vi "Save last shot data.vi"() -> ()   [LabVIEW 2015]
uses:
  Shot data.ctl
  <vilib>/Utility/config.llb/Write Key (I32).vi
  <vilib>/Utility/config.llb/Write Key (String).vi
  <vilib>/Utility/config.llb/Write Key (Double).vi
  <vilib>/Utility/config.llb/NI_LVConfig.lvlib
  <vilib>/Utility/config.llb/Write Key (Boolean).vi
panel:
  out "output 1":timestamp
  out "date/time string":string
  out "time string":string
  out "date string":string
  out "Array":u32[](array[numeric])
  out "Shot data elements":string[](array[string])=["Shot number", "Time", "Magnet ID", "User", "Cell number", "Requested field", "Field direction", "Number of bank frames", "Crowbar resistance, mOhm", "Magnet resistance, mOhm", "Charger voltage, kV", "Frame voltage, kV"]
  in  "Shot data":T1
  in  "File path":path=path "C:/data/LastShot.txt"
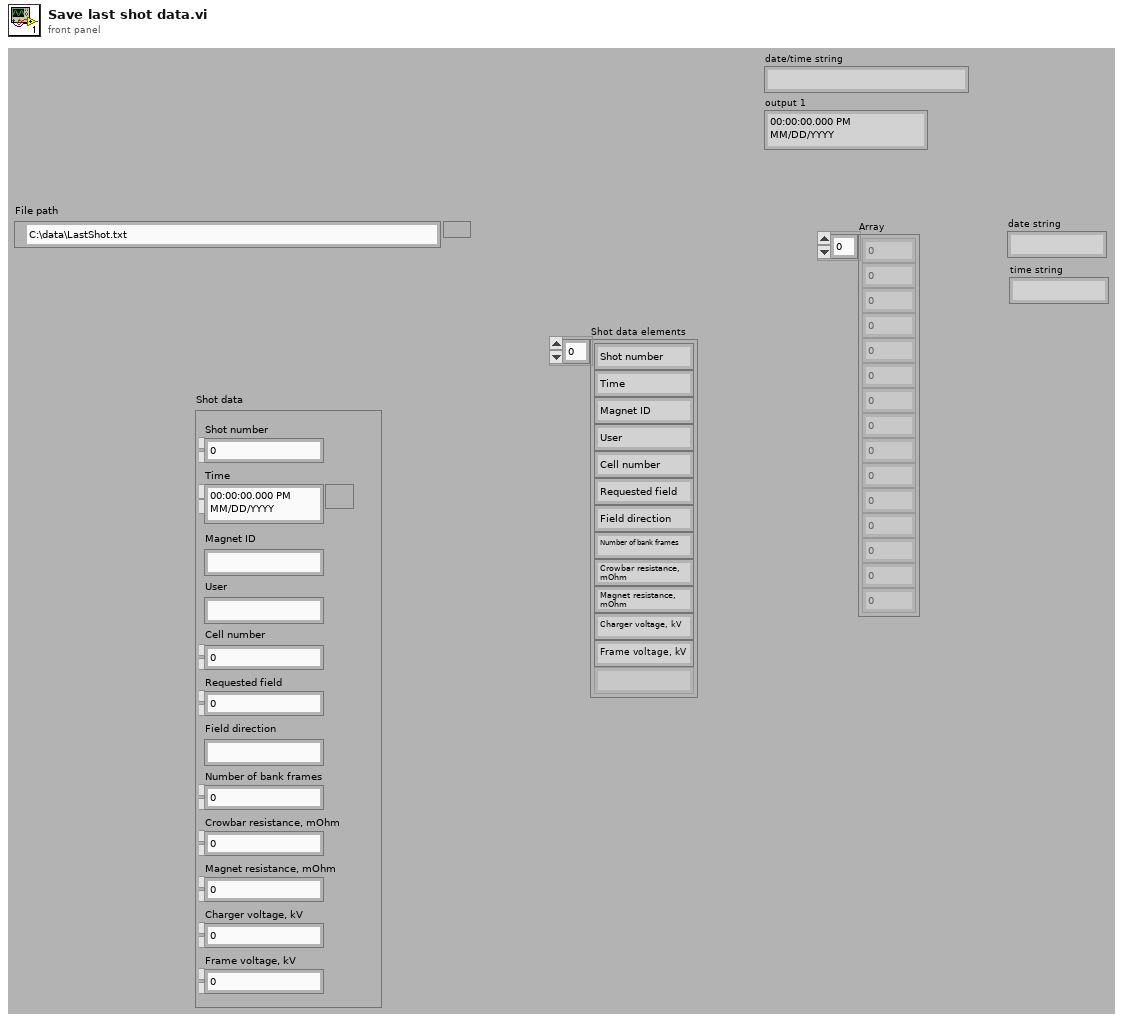
[diagram p1: front panel]
types:
  T1 = typedef "Shot data.ctl" = cluster{"Shot number":i32, "Time":timestamp, "Magnet ID":string, "User":string, "Cell number":i32, "Requested field":dbl, "Field direction":string, "Number of bank frames":i32, "Crowbar resistance, mOhm":dbl, "Magnet resistance, mOhm":dbl, "Charger voltage, kV":dbl, "Frame voltage, kV":dbl}
  T2 = cluster{"Shot data elements[0]":string, "Shot data elements[1]":string, "Shot data elements[2]":string, "Shot data elements[3]":string, "Shot data elements[4]":string, "Shot data elements[5]":string, "Shot data elements[6]":string, "Shot data elements[7]":string, "Shot data elements[8]":string, "Shot data elements[9]":string, "Shot data elements[10]":string, "Shot data elements[11]":string}
  T3 = typedef "NI_LVConfig.lvlib/Config Data RefNum.ctl" = refnum<k1>
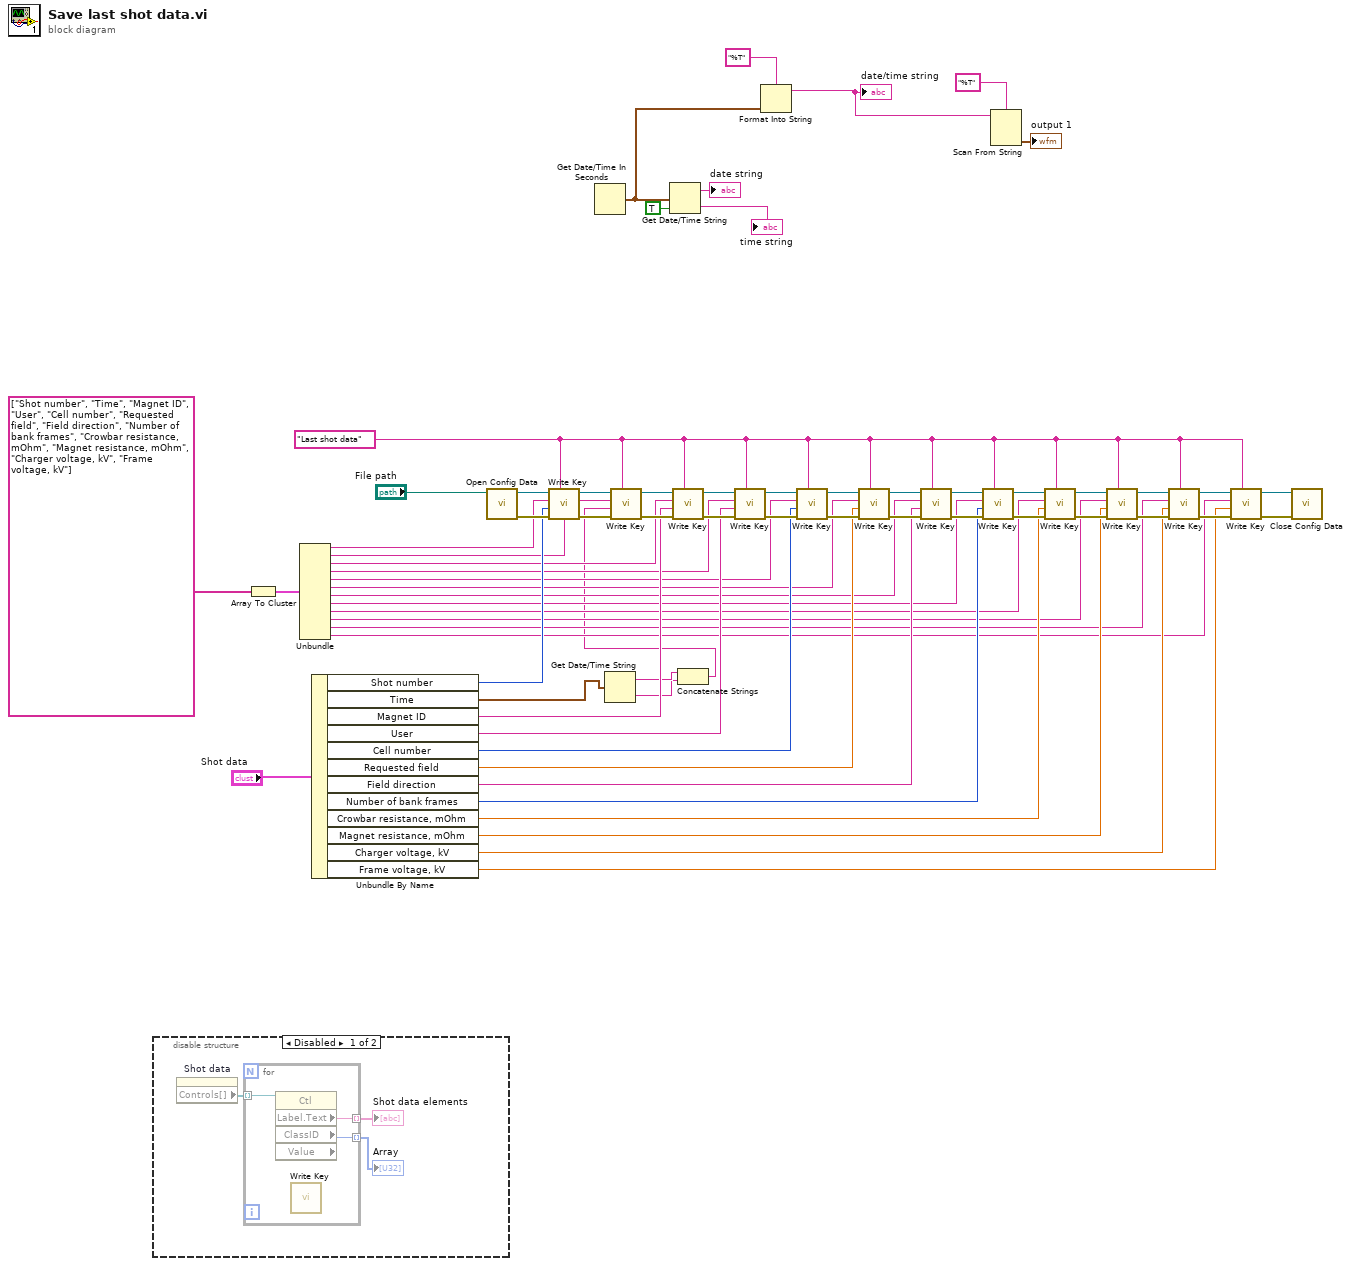
[diagram p0: block diagram]
diagram:
  w35 = "Last shot data" ("section")
  n1 = disable-structure shown="Disabled" {
    frame Disabled {
      n2 = property on="Shot data" class="Clust (strict)"() -> ("Controls[]"=w69:refnum<vi>[])  [unwired: 2 in, 2 out]
      n3 = for {
        tunnel: w69 -> [w72] mode=indexing
        tunnel: [w71] -> w68 mode=indexing
        tunnel: [w70] -> w67 mode=indexing
        n4 = property class="Ctl" props=["Label", "Text", "ClassID", "Value"](reference=w72) -> ("Label.Text"=w71:string, "ClassID"=w70:u32)  [unwired: 1 in, 3 out]
        n5 = call-poly <vilib>:"Write Key.vi"() -> ()  [unwired: 9 in, 3 out]
      }
      "Shot data elements" <- w68
      "Array" <- w67
    }
    frame Enabled {
    }
  }
  n6 = Array To Cluster(array=string[] ["Shot number", "Time", "Magnet ID", "User", "Cell number", "Requested field", "Field direction", "Number of bank frames", "Crowbar resistance, mOhm", "Magnet resistance, mOhm", "Charger voltage, kV", "Frame voltage, kV"] ("Shot data elements")) -> (cluster=w62:T2)
  n7 = Unbundle(w62) -> ("Shot data elements[0]"=w61:string, "Shot data elements[1]"=w40:string, "Shot data elements[2]"=w24:string, "Shot data elements[3]"=w23:string, "Shot data elements[4]"=w22:string, "Shot data elements[5]"=w21:string, "Shot data elements[6]"=w20:string, "Shot data elements[7]"=w19:string, "Shot data elements[8]"=w18:string, "Shot data elements[9]"=w17:string, "Shot data elements[10]"=w16:string, "Shot data elements[11]"=w15:string)
  n8 = Unbundle By Name("Shot data") -> ("Shot number"=w59:i32, "Time"=w2:timestamp, "Magnet ID"=w34:string, "User"=w33:string, "Cell number"=w32:i32, "Requested field"=w31:dbl, "Field direction"=w30:string, "Number of bank frames"=w29:i32, "Crowbar resistance, mOhm"=w28:dbl, "Magnet resistance, mOhm"=w27:dbl, "Charger voltage, kV"=w26:dbl, "Frame voltage, kV"=w25:dbl)
  n9 = call <vilib>:"Open Config Data.vi"("configuration file path"="File path") -> ("error out"=w64:errorcluster, "refnum"=w65:T3)  [unwired: 8 in, 1 out]
  n10 = call-poly <vilib>:"Write Key.vi"("section"=w35, "error in (no error)"=w64, "value"=w59, "key"=w61, "refnum"=w65) -> ("error out"=w42:errorcluster, "refnum out"=w41:T3)  [unwired: 4 in, 1 out]
  n11 = Get Date/Time In Seconds() -> (seconds since 1Jan1904=w6:timestamp)
  n12 = Get Date/Time String(seconds (now)=w2) -> (date string=w4:string, time string=w3:string)  [unwired: 2 in]
  n13 = Get Date/Time String(seconds (now)=w6, want seconds? (F)=TRUE) -> (date string=→"date string":string, time string=→"time string":string)  [unwired: 1 in]
  n14 = Concatenate Strings(w4, w3) -> (w1:string)
  n15 = call-poly <vilib>:"Write Key.vi"("section"=w35, "error in (no error)"=w42, "value"=w1, "key"=w40, "refnum"=w41) -> ("error out"=w44:errorcluster, "refnum out"=w43:T3)  [unwired: 4 in, 1 out]
  n16 = call-poly <vilib>:"Write Key.vi"("section"=w35, "error in (no error)"=w44, "value"=w34, "key"=w24, "refnum"=w43) -> ("error out"=w45:errorcluster, "refnum out"=w46:T3)  [unwired: 4 in, 1 out]
  n17 = call-poly <vilib>:"Write Key.vi"("section"=w35, "error in (no error)"=w45, "value"=w33, "key"=w23, "refnum"=w46) -> ("error out"=w48:errorcluster, "refnum out"=w47:T3)  [unwired: 4 in, 1 out]
  n18 = Format Into String(format string="%T", w6) -> (resulting string=w5:string)  [unwired: 2 in, 1 out]
  "date/time string" <- w5
  n19 = call-poly <vilib>:"Write Key.vi"("section"=w35, "error in (no error)"=w48, "value"=w32, "key"=w22, "refnum"=w47) -> ("error out"=w49:errorcluster, "refnum out"=w50:T3)  [unwired: 4 in, 1 out]
  n20 = call-poly <vilib>:"Write Key.vi"("section"=w35, "error in (no error)"=w49, "value"=w31, "key"=w21, "refnum"=w50) -> ("error out"=w39:errorcluster, "refnum out"=w38:T3)  [unwired: 4 in, 1 out]
  n21 = call-poly <vilib>:"Write Key.vi"("section"=w35, "error in (no error)"=w39, "value"=w30, "key"=w20, "refnum"=w38) -> ("error out"=w52:errorcluster, "refnum out"=w51:T3)  [unwired: 4 in, 1 out]
  n22 = call-poly <vilib>:"Write Key.vi"("section"=w35, "error in (no error)"=w52, "value"=w29, "key"=w19, "refnum"=w51) -> ("error out"=w53:errorcluster, "refnum out"=w54:T3)  [unwired: 4 in, 1 out]
  n23 = Scan From String(format string="%T", input string=w5) -> (output 1=→"output 1":timestamp)  [unwired: 3 in, 3 out]
  n24 = call-poly <vilib>:"Write Key.vi"("section"=w35, "error in (no error)"=w53, "value"=w28, "key"=w18, "refnum"=w54) -> ("error out"=w56:errorcluster, "refnum out"=w55:T3)  [unwired: 4 in, 1 out]
  n25 = call-poly <vilib>:"Write Key.vi"("section"=w35, "error in (no error)"=w56, "value"=w27, "key"=w17, "refnum"=w55) -> ("error out"=w57:errorcluster, "refnum out"=w58:T3)  [unwired: 4 in, 1 out]
  n26 = call-poly <vilib>:"Write Key.vi"("section"=w35, "error in (no error)"=w57, "value"=w26, "key"=w16, "refnum"=w58) -> ("error out"=w37:errorcluster, "refnum out"=w36:T3)  [unwired: 4 in, 1 out]
  n27 = call-poly <vilib>:"Write Key.vi"("section"=w35, "error in (no error)"=w37, "value"=w25, "key"=w15, "refnum"=w36) -> ("error out"=w14:errorcluster, "refnum out"=w13:T3)  [unwired: 4 in, 1 out]
  n28 = call <vilib>:"Close Config Data.vi"("error in (no error)"=w14, "refnum"=w13) -> ()  [unwired: 8 in, 2 out]
